vi "Cnt.vi"(6 "n-1":i32=319, 8 "inc":i32=40) -> (0 "i":i32, 4 "end":bool)   [LabVIEW 2015]
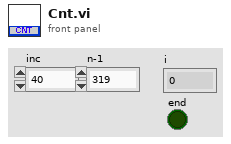
[diagram p1: front panel]
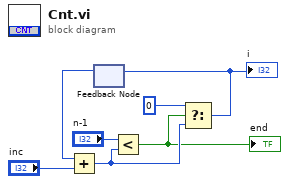
[diagram p0: block diagram]
diagram:
  n1 = feedback #1() -> (w4:i32)  [unwired: 1 in]
  n2 = Add(x=w4, y="inc") -> (x+y=w6:i32)
  n3 = Less?(x="n-1", y=w6) -> (x < y?=w2:bool)
  "end" <- w2
  n4 = Select(t=0 ("index"), s=w2, f=w6) -> (s? t:f=w7:i32)
  "i" <- w7
  n5 = feedback-in #1(w7) -> ()
